vi "GV PhotocounterInputSelector.vi"() -> ()   [LabVIEW 2017]
panel:
  out "PhotocounterInputSelector":bool
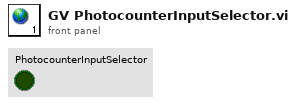
[diagram p1: front panel]
diagram:
